vi "MakeOperationalCycleMacro.vi"(11 "TestCycleParameters":T1={"TAmb"=20.0, "HeaterTestTemp"=-80.0, "HeaterTestDwell(min)"=30, "HeaterTestDuration"=15, "MinOpTemp"=-50.0, "MinOpDwell(min)"=30, "TestHeatingRate (deg/min)"=0.4, "SurviveCycleParameters"={"MinSurviveTemp"=-131.5, "MinSurvive Dwell(min)"=10, "MaxSurviveTemp"=50.0, "MaxSurviveDwell(min)"=30, "ControlInput"=2, "ColdStandOff"=4.0, "HotStandoff"=5.0, "SteadyPWM"=20, "MaxCoolingRate (deg/min)"=3.75, "MaxHeatingRate (deg/min)"=2.5}, "CycleType"=0, "MaxOpTemp"=-50.0, "MaxOpDwell(min)"=30} {"CycleType" items=["Survival", "Operational"]; "SurviveCycleParameters"."SteadyPWM" min=0 max=100 step=1; "SurviveCycleParameters"."ControlInput" items=["3A", "3B", "3C", "3D", "4A", "4B", "4C", "4D"]}) -> (1 "Profile":cluster{dbl[], dbl[]}(graph)={[0.0, 25.0, 85.0, 97.5, 127.5, 142.5, 150.0, 180.0, 430.0, 460.0], [20.0, -130.0, -130.0, -80.0, -80.0, -80.0, -50.0, -50.0, 50.0, 50.0]}, 3 "resulting string":string="define onecycle (pwm=100 run pwmloop 5A.PID.Ramp=0 5A.PID.SetPoint=-130.0 5A.PID.input=3A while(#3A>-180.0){pause 0.2 s}  pwm=-50 pause 60 min pwm=0 5A.PID.SetPoint=-80.000000 while(#3A<-30.000000)(pause 0.2 s} pwm=-50 pause 45 min pwm=0 5A.PID.SetPoint=-50.000000 while(#3A<0.000000){pause 0.2 s} pwm=-50 pause 30 5A.PID.Ramp=0.006667 5A.PID.SetPoint=50.000000 while (#3A<100.000000){pause 0.2 s} pause 30 min kill pwmloop)\n")   [LabVIEW 2024]
uses:
  controls/TestCycleParams.ctl
  controls/SurviveCycleParams.ctl
  controls/ControlInput.ctl
panel:
  in  "Tab Control":enum32{"RampProfile", "PTC Code"}(tab)
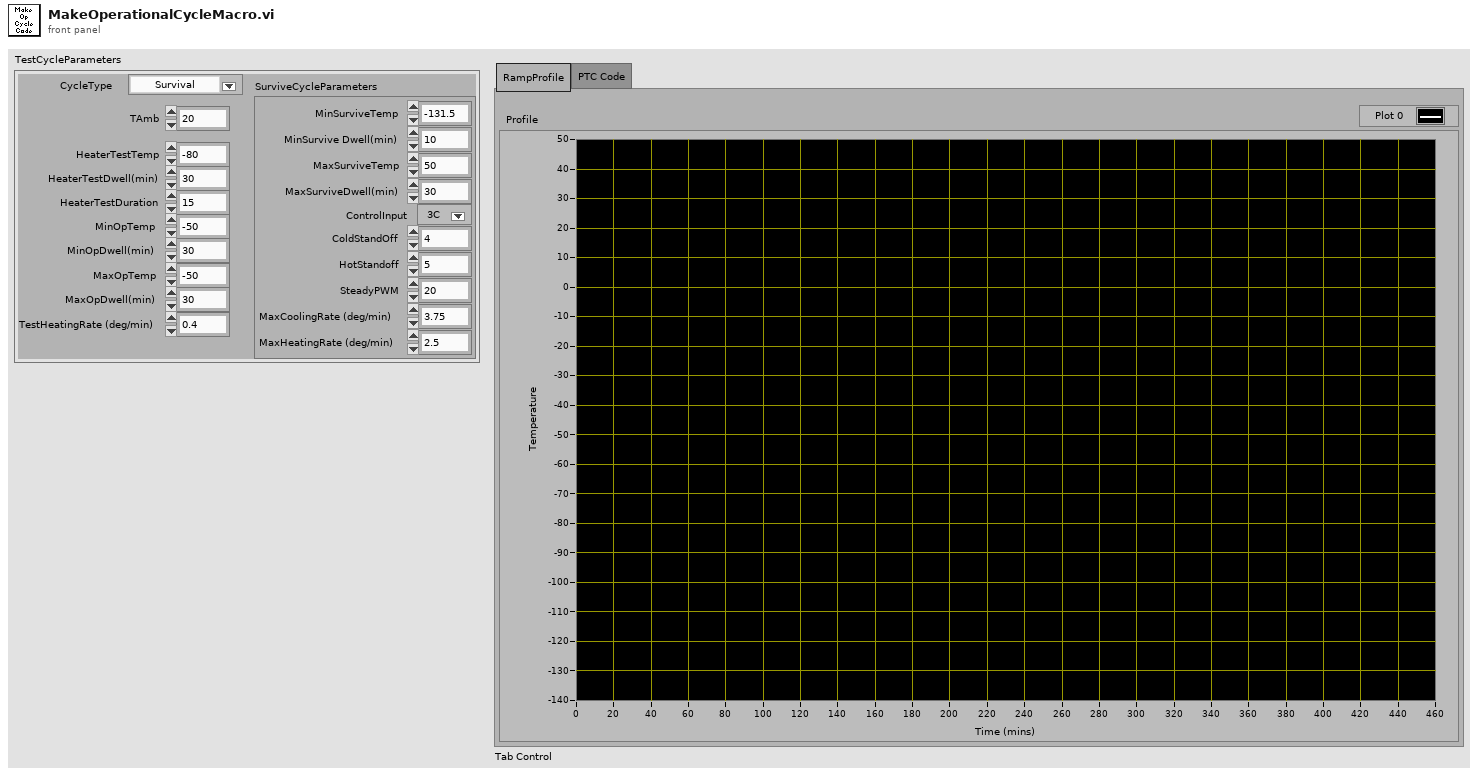
[diagram p1: front panel]
types:
  T1 = typedef "TestCycleParams.ctl" = cluster{"TAmb":dbl, "HeaterTestTemp":dbl, "HeaterTestDwell(min)":i32, "HeaterTestDuration":i32, "MinOpTemp":dbl, "MinOpDwell(min)":i32, "TestHeatingRate (deg/min)":dbl, "SurviveCycleParameters":T2, "CycleType":u16, "MaxOpTemp":dbl, "MaxOpDwell(min)":i32}
  T2 = typedef "SurviveCycleParams.ctl" = cluster{"MinSurviveTemp":dbl, "MinSurvive Dwell(min)":i32, "MaxSurviveTemp":dbl, "MaxSurviveDwell(min)":i32, "ControlInput":T3, "ColdStandOff":dbl, "HotStandoff":dbl, "SteadyPWM":i32, "MaxCoolingRate (deg/min)":dbl, "MaxHeatingRate (deg/min)":dbl}
  T3 = typedef "ControlInput.ctl" = u16
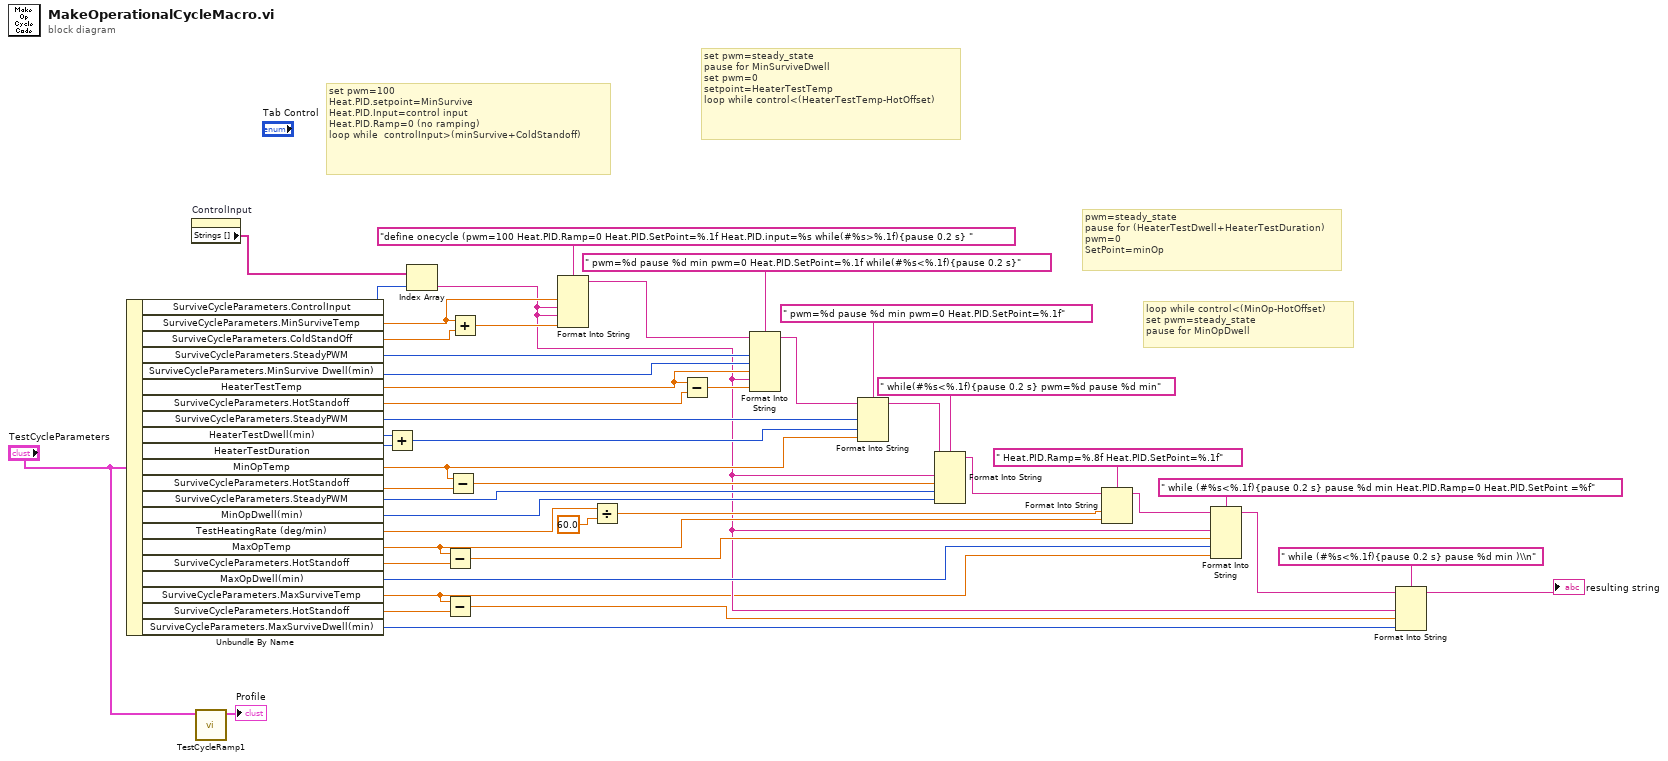
[diagram p0: block diagram]
diagram:
  # "loop while control<(MinOp-HotOffset)\nset pwm=steady_state\npause for MinOpDwell"
  # "pwm=steady_state\npause for (HeaterTestDwell+HeaterTestDuration)\npwm=0\nSetPoint=minOp"
  # "set pwm=steady_state\npause for MinSurviveDwell\nset pwm=0\nsetpoint=HeaterTestTemp\nloop while control<(HeaterTestTemp-HotOffset)"
  # "set pwm=100\nHeat.PID.setpoint=MinSurvive\nHeat.PID.Input=control input\nHeat.PID.Ramp=0 (no ramping)\nloop while  controlInput>(minSurvive+ColdStandoff)"
  n1 = Unbundle By Name("TestCycleParameters") -> ("SurviveCycleParameters.ControlInput"=w12:T3, "SurviveCycleParameters.MinSurviveTemp"=w40:dbl, "SurviveCycleParameters.ColdStandOff"=w39:dbl, "SurviveCycleParameters.SteadyPWM"=w33:i32, "SurviveCycleParameters.MinSurvive Dwell(min)"=w34:i32, "HeaterTestTemp"=w35:dbl, "SurviveCycleParameters.HotStandoff"=w37:dbl, "SurviveCycleParameters.SteadyPWM"=w36:i32, "HeaterTestDwell(min)"=w31:i32, "HeaterTestDuration"=w29:i32, "MinOpTemp"=w28:dbl, "SurviveCycleParameters.HotStandoff"=w27:dbl, "SurviveCycleParameters.SteadyPWM"=w25:i32, "MinOpDwell(min)"=w24:i32, "TestHeatingRate (deg/min)"=w22:dbl, "MaxOpTemp"=w9:dbl, "SurviveCycleParameters.HotStandoff"=w8:dbl, "MaxOpDwell(min)"=w14:i32, "SurviveCycleParameters.MaxSurviveTemp"=w4:dbl, "SurviveCycleParameters.HotStandoff"=w3:dbl, "SurviveCycleParameters.MaxSurviveDwell(min)"=w1:i32)
  n2 = property on="ControlInput" class="Ring (strict)"() -> ("Strings []"=w10:string[])  [unwired: 2 in, 2 out]
  n3 = call "TestCycleRamp1.vi"("TestCycleParameters"="TestCycleParameters") -> ("Profile"=→"Profile":cluster{dbl[], dbl[]})  [unwired: 10 in]
  n4 = Add(x=w31, y=w29) -> (x+y=w30:i32)
  n5 = Index Array(array=w10, index=w12) -> (element=w5:string)
  n6 = Subtract(x=w9, y=w8) -> (x-y=w15:dbl)
  n7 = Subtract(x=w4, y=w3) -> (x-y=w2:dbl)
  n8 = Subtract(x=w28, y=w27) -> (x-y=w26:dbl)
  n9 = Add(x=w40, y=w39) -> (x+y=w38:dbl)
  n10 = Format Into String(format string="define onecycle (pwm=100 Heat.PID.Ramp=0 Heat.PID.SetPoint=%.1f Heat.PID.input=%s while(#%s>%.1f){pause 0.2 s} ", w40, w5, w5, w38) -> (resulting string=w42:string)  [unwired: 2 in, 1 out]
  n11 = Divide(x=w22, y=60.0) -> (x/y=w20:dbl)
  n12 = Subtract(x=w35, y=w37) -> (x-y=w32:dbl)
  n13 = Format Into String(format string=" pwm=%d pause %d min pwm=0 Heat.PID.SetPoint=%.1f while(#%s<%.1f){pause 0.2 s}", initial string=w42, w33, w34, w35, w5, w32) -> (resulting string=w43:string)  [unwired: 1 in, 1 out]
  n14 = Format Into String(format string=" pwm=%d pause %d min pwm=0 Heat.PID.SetPoint=%.1f", initial string=w43, w36, w30, w28) -> (resulting string=w41:string)  [unwired: 1 in, 1 out]
  n15 = Format Into String(format string=" while(#%s<%.1f){pause 0.2 s} pwm=%d pause %d min", initial string=w41, w5, w26, w25, w24) -> (resulting string=w19:string)  [unwired: 1 in, 1 out]
  n16 = Format Into String(format string=" Heat.PID.Ramp=%.8f Heat.PID.SetPoint=%.1f", initial string=w19, w20, w9) -> (resulting string=w18:string)  [unwired: 1 in, 1 out]
  n17 = Format Into String(format string=" while (#%s<%.1f){pause 0.2 s} pause %d min Heat.PID.Ramp=0 Heat.PID.SetPoint =%f", initial string=w18, w5, w15, w14, w4) -> (resulting string=w17:string)  [unwired: 1 in, 1 out]
  n18 = Format Into String(format string=" while (#%s<%.1f){pause 0.2 s} pause %d min )\\n", initial string=w17, w5, w2, w1) -> (resulting string=→"resulting string":string)  [unwired: 1 in, 1 out]
